vi "Set Master-Slave Jog Velocity Scalling Coefficients.vi"(4 "error in (no error)":errorcluster, 5 "B (0)":dbl min=0.0 format="%.6g", 6 "A (0)":dbl min=0.0 format="%.6g", 7 "VISA resource name":refnum<visa-resource-name>) -> (0 "error out":errorcluster, 3 "VISA resource name out":refnum<visa-resource-name>)   [LabVIEW 2015, in "Newport ESP301.lvlib"]
doc: "This command sets the jog velocity scaling coefficients for slave axis. The jog velocity of slave axis is computed once every interval using user specified scaling coefficients and the master axis velocity at the time of computation. The user specified coefficients are used as follows:\nd(x(s))/dt = A.d(x((m))/dt + B.(d(x(m))/dt)^2.sgn(d(x((m))/dt)\nwhere d(x(s))/dt is the jog velocity of the slave and d(x((m))/dt is the velocity of the master axis.\nRefer SI command to specify slave jog velocity update interval.\n<B>Note:</B> Appropriate trajectory mode has to be specified using TJ command before this command becomes effective."
uses:
  Newport ESP301.lvlib
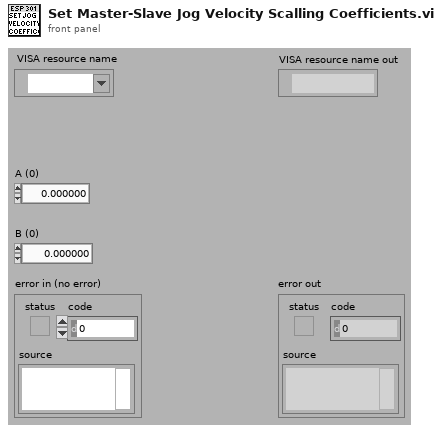
[diagram p1: front panel]
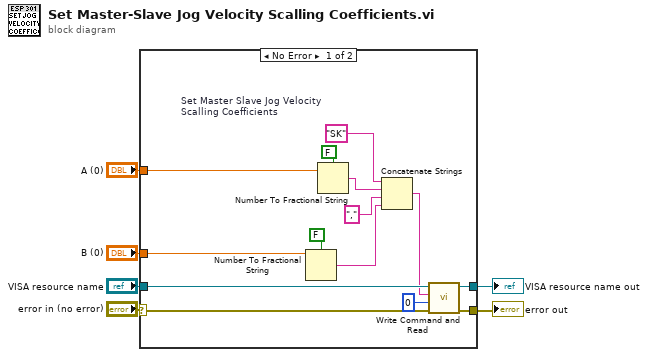
[diagram p0: block diagram]
diagram:
  n1 = case shown="No Error" "error in (no error)" {
    selector: "error in (no error)" -> [w17 w22]
    tunnel: [w19 w22] -> w6
    tunnel: "VISA resource name" -> [w20 w21]
    tunnel: [w18 w21] -> w5
    tunnel: "A (0)" -> [w12 _]
    tunnel: "B (0)" -> [w13 _]
    frame No Error {
      w16 = "SK"  # Set Master Slave Jog Velocity Scalling Coefficients
      n2 = Number To Fractional String(use system decimal point (T)=FALSE ("utiliser le séparateur décimal du système (V)"), number=w13) -> (F-format string=w7:string)  [unwired: 2 out]
      n3 = Number To Fractional String(use system decimal point (T)=FALSE ("utiliser le séparateur décimal du système (V)"), number=w12) -> (F-format string=w9:string)  [unwired: 2 in]
      n4 = Concatenate Strings(w16, w9, "," ("chaîne"), w7) -> (w15:string)
      n5 = call "Write Command and Read.vi"("error in (no error)"=w17, "Bytes to read (100)"=u32 0, "Command"=w15, "VISA resource name"=w20) -> ("error out"=w19:errorcluster, "VISA resource name out"=w18:refnum<visa-resource-name>)  [unwired: 3 in, 1 out]
    }
    frame Error {
    }
  }
  "error out" <- w6
  "VISA resource name out" <- w5
